vi "tem.vi"() -> ()   [LabVIEW 2020]
panel:
  out "fahrenheit":dbl(slide) scale=0.0..100.0
  out "celsius":dbl(slide) scale=0.0..100.0
  out "fahrenheit":dbl
  in  "celsius":dbl
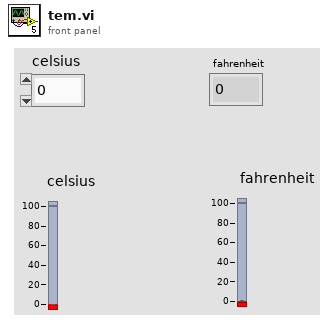
[diagram p1: front panel]
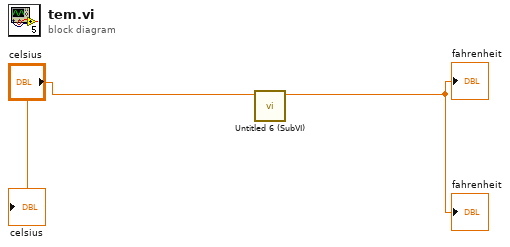
[diagram p0: block diagram]
diagram:
  n1 = call "Untitled 6 (SubVI).vi"("celsius"="celsius") -> ("Numeric"=→"fahrenheit" →"fahrenheit":dbl)  [unwired: 10 in]
  "celsius" <- "celsius"
